vi "GetText.vi"(8 "error in":errorcluster, 11 "Central Error Handler editor node in":refnum<class "Central Error Handler editor node.lvclass">) -> (0 "error out":errorcluster, 1 "additional text":string, 2 "text":string, 3 "Central Error Handler editor node out":refnum<class "Central Error Handler editor node.lvclass">, 4 "glyph":string)   [LabVIEW 2017, in "Central Error Handler editor node.lvclass"]
uses:
  Central Error Handler editor node.lvclass
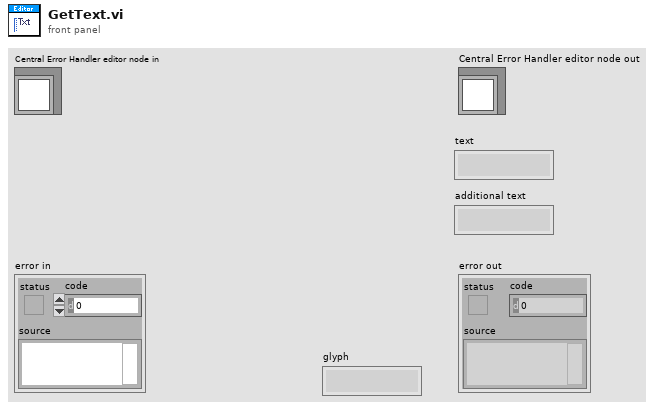
[diagram p1: front panel]
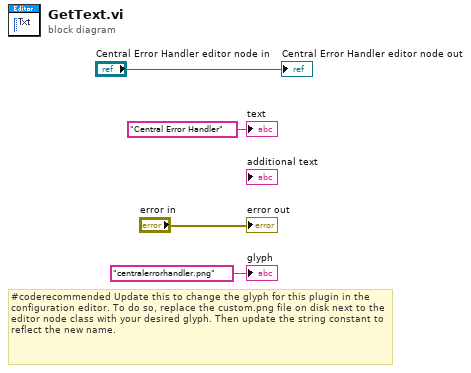
[diagram p0: block diagram]
diagram:
  # "#coderecommended Update this to change the glyph for this plugin in the configuration editor. To do so, replace the custom.png file on disk next to the editor node class with your desired glyph. Then update the string constant to reflect the new name."
  "error out" <- "error in"
  "Central Error Handler editor node out" <- "Central Error Handler editor node in"
  "text" <- "Central Error Handler" ("text")
  "glyph" <- "centralerrorhandler.png" ("glyph")
